vi "Node.vi"(8 "error in (no error)":errorcluster, 11 "Task in":refnum<class "Task Config.lvclass">) -> (0 "error out":errorcluster, 2 "Node":refnum<class "Node Config.lvclass">, 3 "Task out":refnum<class "Task Config.lvclass">)   [LabVIEW 2020, in "VolatusConfig.lvlib" / "Task Config.lvclass"]
uses:
  Task Config.lvclass
  C:/dev/lv20CE/relink/lv-volatus/VolatusConfig/VolatusConfigElement/VolatusConfigElement.lvclass
  Node/Node Config.lvclass
  Meta Type.ctl
  VolatusConfigElement/VolatusConfigElement.lvclass/VolatusConfigElement.ctl
  VolatusConfigElement/Element.vi
  lv-cdm/CDM-Config/Config Lookup/Match Meta.vi
  lv-cdm/CDM-Config/Config Element/Owner.vi
  lv-cdm/CDM-Config/Config Filter/Config Lookup.lvclass
  Task Config.lvclass/Task Config.ctl
  VolatusConfigElement/VolatusConfigElement.lvclass
  VolatusConfig.lvlib
  C:/dev/lv20CE/relink/lv-volatus/VolatusConfig/Task/Task Config.lvclass
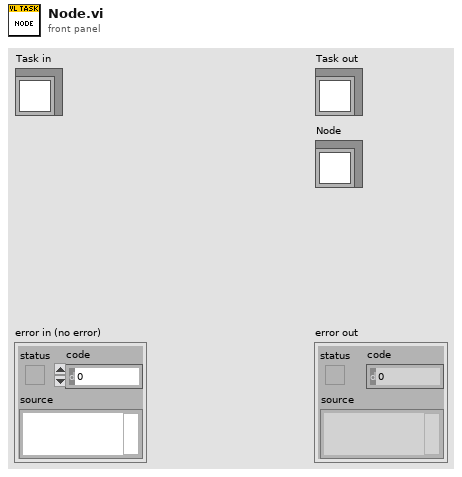
[diagram p1: front panel]
types:
  T1 = typedef "VolatusConfig.lvlib/Meta Type.ctl" = enum16{"UNKNOWN", "VL_System", "VL_Cluster", "VL_Node", "VL_Task", "VL_Group", "VL_Channel", "VL_Task_List", "VL_Scaling", "VL_Sensor", "VL_Sensor_List", "VL_Scale"}
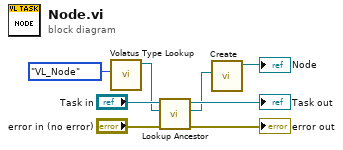
[diagram p0: block diagram]
diagram:
  n1 = call "Volatus Type Lookup.vi"("Meta Type"=Meta_Type."VL_Node") -> ("Config Lookup out"=w4:refnum<class "Config Lookup.lvclass">)  [unwired: 9 in, 1 out]
  n2 = call "Lookup Ancestor.vi"("error in (no error)"="error in (no error)", "Lookup"=w4, "VolatusConfigElement in"="Task in") -> ("error out"=→"error out":errorcluster, "Ancestor"=w2:refnum<class "Config Element.lvclass">, "VolatusConfigElement out"=→"Task out":refnum<class "Task Config.lvclass">)  [unwired: 6 in]
  n3 = call "Create.vi"("Element"=w2) -> ("Node out"=→"Node":refnum<class "Node Config.lvclass">)  [unwired: 9 in, 1 out]
